vi "Configure Marker Search.vi"(7 "Marker Search (Max Peak)":T1, 8 "error in (no error)":errorcluster, 10 "Marker Number (1)":u32=1 min=1, 11 "MXA in":refnum<class "MXA.lvclass">) -> (0 "error out":errorcluster, 3 "MXA out":refnum<class "MXA.lvclass">)   [LabVIEW 2020, in "MXA.lvclass"]
uses:
  MXA.lvclass
  C:/Sandbox/RF Bench/Source Code/WiSpry Test Framework/Instruments/Instrument.lvclass
  Controls/Marker Search.ctl
  Instrument.lvclass/Instrument.ctl
  Instrument.lvclass
  <instrlib>/Agilent MXA Series/Agilent MXA Series.lvlib
  Spectrum Analyzer.lvclass
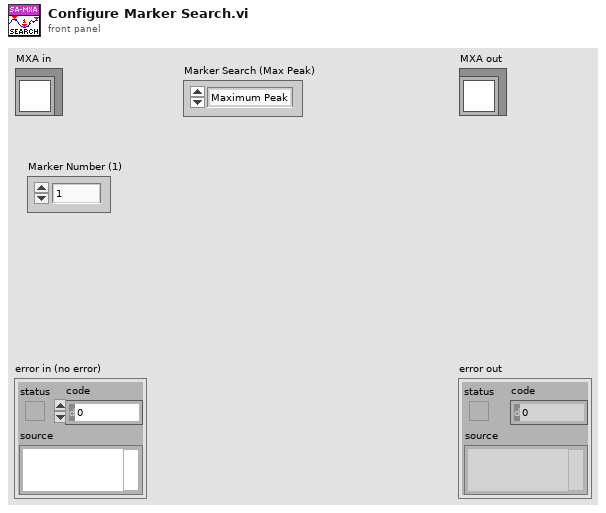
[diagram p1: front panel]
types:
  T1 = typedef "Spectrum Analyzer.lvclass/Marker Search.ctl" = enum16{"Maximum Peak", "Maximum Next", "Maximum Right", "Maximum Left", "Minimum Peak", "Minimum Next", "Minimum Right", "Minimum Left"}
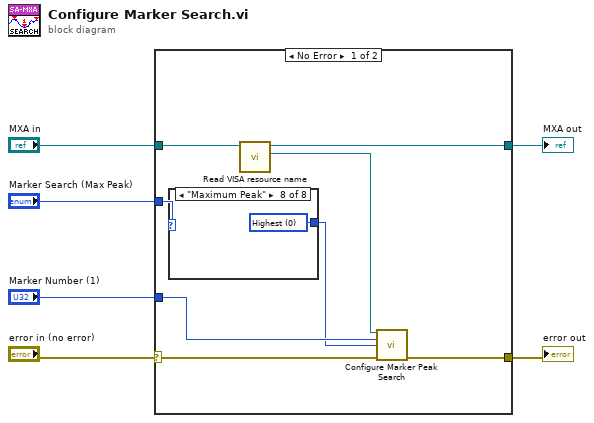
[diagram p0: block diagram]
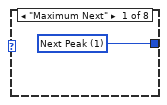
[diagram p2: hidden frame]
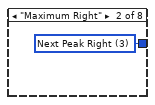
[diagram p3: hidden frame]
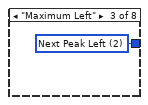
[diagram p4: hidden frame]
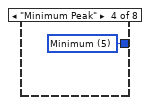
[diagram p5: hidden frame]
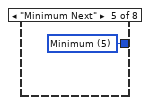
[diagram p6: hidden frame]
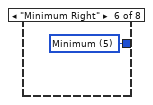
[diagram p7: hidden frame]
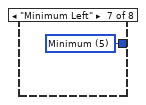
[diagram p8: hidden frame]
diagram:
  n1 = case shown="No Error" "error in (no error)" {
    selector: "error in (no error)" -> [w10 w24]
    tunnel: "MXA in" -> [w14 w23]
    tunnel: [w9 w24] -> w5
    tunnel: [w13 w23] -> w4
    tunnel: "Marker Number (1)" -> [w11 _]
    tunnel: "Marker Search (Max Peak)" -> [w8 _]
    frame No Error {
      n2 = case shown="\"Maximum Peak\"" w8 {
        tunnel: [w15 w16 w17 w18 w19 w20 w21 w22] -> w7
        frame "Maximum Next" {
          w15 = 1 items=["Highest", "Next Peak", "Next Peak Left", "Next Peak Right", "Pk-Pk Search", "Minimum"] ("Marker Search (0: Highest)")
        }
        frame "Maximum Right" {
          w16 = 3 items=["Highest", "Next Peak", "Next Peak Left", "Next Peak Right", "Pk-Pk Search", "Minimum"] ("Marker Search (0: Highest)")
        }
        frame "Maximum Left" {
          w17 = 2 items=["Highest", "Next Peak", "Next Peak Left", "Next Peak Right", "Pk-Pk Search", "Minimum"] ("Marker Search (0: Highest)")
        }
        frame "Minimum Peak" {
          w18 = 5 items=["Highest", "Next Peak", "Next Peak Left", "Next Peak Right", "Pk-Pk Search", "Minimum"] ("Marker Search (0: Highest)")
        }
        frame "Minimum Next" {
          w19 = 5 items=["Highest", "Next Peak", "Next Peak Left", "Next Peak Right", "Pk-Pk Search", "Minimum"] ("Marker Search (0: Highest)")
        }
        frame "Minimum Right" {
          w20 = 5 items=["Highest", "Next Peak", "Next Peak Left", "Next Peak Right", "Pk-Pk Search", "Minimum"] ("Marker Search (0: Highest)")
        }
        frame "Minimum Left" {
          w21 = 5 items=["Highest", "Next Peak", "Next Peak Left", "Next Peak Right", "Pk-Pk Search", "Minimum"] ("Marker Search (0: Highest)")
        }
        frame "Maximum Peak" {
          w22 = 0 items=["Highest", "Next Peak", "Next Peak Left", "Next Peak Right", "Pk-Pk Search", "Minimum"] ("Marker Search (0: Highest)")
        }
      }
      n3 = call "Read VISA resource name.vi"("Instrument in"=w14) -> ("VISA resource name"=w12:refnum<visa-resource-name>, "Instrument out"=w13:refnum<class "MXA.lvclass">)  [unwired: 9 in]
      n4 = call <instrlib>:"Configure Marker Peak Search.vi"("VISA resource name"=w12, "Active Marker (1: Marker1)"=w11, "Marker Search (0: Highest)"=w7, "error in (no error)"=w10) -> ("error out"=w9:errorcluster)  [unwired: 10 in, 1 out]
    }
    frame Error {
    }
  }
  "error out" <- w5
  "MXA out" <- w4
